vi "_PC_RTFunc_ReadRTTimeStamp.vi"(8 "error in (no error)":errorcluster) -> (0 "error out":errorcluster, 1 "64bit integer":i64, 2 "RT_SysTimeStamp":timestamp)   [LabVIEW 2018]
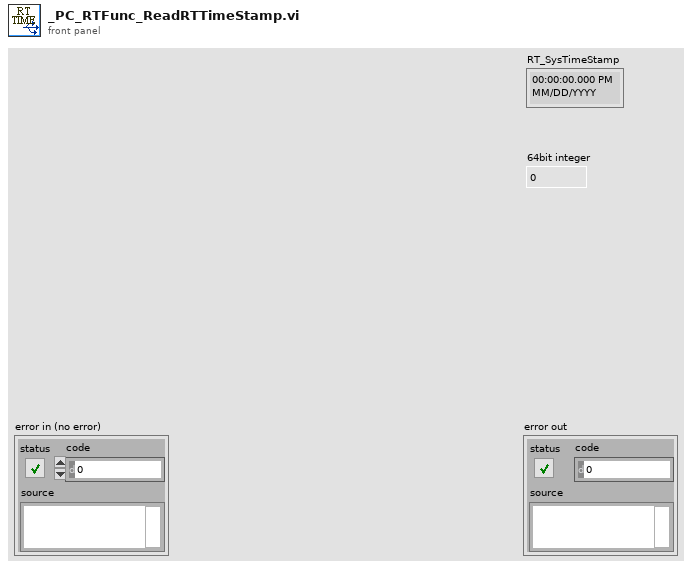
[diagram p1: front panel]
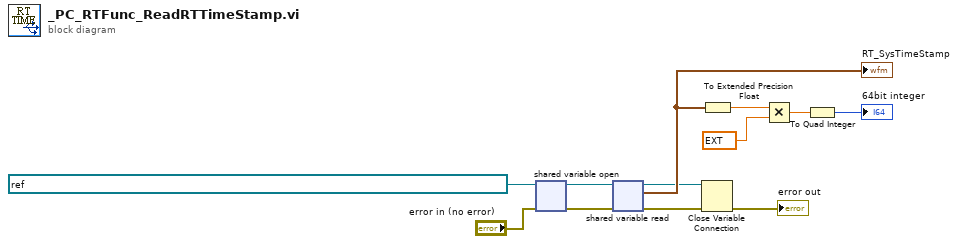
[diagram p0: block diagram]
diagram:
  n1 = shared-variable-open(refnum<k21> "ni.var.psp://NI-sbRIO/_RT_CtrlLoop_ResourcesMonitor_Variables/RT_SysTimeStamp" ("shared variable refnum in"), "error in (no error)") -> (w6:refnum<k21>, w5:errorcluster)
  n2 = shared-variable-read(w6, w5) -> (w3:refnum<k21>, w2:errorcluster, w12:timestamp)
  "RT_SysTimeStamp" <- w12
  n3 = Close Variable Connection(8:w2, 11:w3) -> (0:→"error out":errorcluster)
  n4 = To Extended Precision Float(1:w12) -> (0:w11:ext)
  n5 = Multiply(x=w11, y=ext 1000.0) -> (x*y=w9:ext)
  n6 = To Quad Integer(1:w9) -> (0:→"64bit integer":i64)
